vi "test BC + RTs.vi"(8 "error in":errorcluster, 11 "TestCase in":refnum<class "Create Execution Unit.lvclass">) -> (0 "error out":errorcluster, 3 "TestCase out":refnum<class "Create Execution Unit.lvclass">)   [LabVIEW 2020, in "Create Execution Unit.lvclass"]
uses:
  Create Execution Unit.lvclass
  C:/Program Files (x86)/National Instruments/LabVIEW 2020/vi.lib/addons/_JKI Toolkits/VI Tester/TestCase.llb/TestCase.lvclass
  Shared/Map of Messages to Value Indexes.ctl
  Shared/Message Map Key.ctl
  Engine/Implementation/Rx Execution Unit/Message Map Value.ctl
  Shared/Message Definition.ctl
  Shared/Message Type.ctl
  Shared/Terminal Endpoint.ctl
  Shared/Address.ctl
  Shared/Parameter Definition.ctl
  <vilib>/addons/_JKI Toolkits/VI Tester/TestCase.llb/TestCase.lvclass
  Scripting/AIM MIL-STD-1553 Scripting.lvlib
  Shared/Initialization Method.ctl
  Shared/Device Parameters.ctl
  Engine/Implementation/Execution Unit Factory/Execution Unit Factory.lvclass
  Engine/Implementation/Rx Execution Unit/Rx Execution Unit.lvclass
  Engine/Implementation/Shared Resources/Shared Resources.lvclass
  Shared/Data Word Format.ctl
  Engine/Custom Device/Logging Configuration.ctl
  Engine/Custom Device/Custom Device.lvlib
  Shared/Coupling Mode.ctl
  Shared/Bus Selection.ctl
  C:/dev/git/niveristand-custom-device-testing-tools/VeriStandScriptingTestCase/VeriStandScriptingTestCase.lvclass
  C:/dev/git/niveristand-aim-milStd1553-custom-device/Source/Custom Device Support/Tests/Unit/Create Execution Unit/Create Execution Unit.lvclass
  C:/dev/git/niveristand-aim-milStd1553-custom-device/Source/Custom Device Support/Engine/Implementation/Shared Resources/Shared Resources.lvclass
  C:/dev/git/niveristand-aim-milStd1553-custom-device/Source/Custom Device Support/Engine/Interfaces/Shared Resources/Shared Resources.lvclass
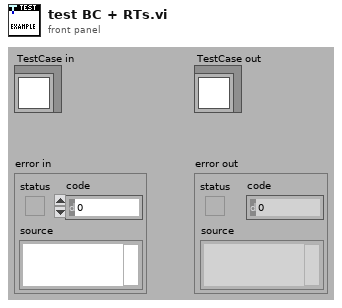
[diagram p1: front panel]
types:
  T1 = typedef "Map of Messages to Value Indexes.ctl" = map{T2, T3}
  T2 = typedef "Message Map Key.ctl" = cluster{"HW channel":u16, "terminal address":u16, "subaddress":u16, "mode code":u16}
  T3 = typedef "AIM MIL-STD-1553 Engine.lvlib/Implementation.lvlib/Rx Execution Unit.lvclass/Message Map Value.ctl" = cluster{"value indexes":i32[], "message":T4, "Tx status count":i32, "Rx status count":i32}
  T4 = typedef "Message Definition.ctl" = cluster{"name":string, "message type":T5, "endpoint Tx":T6, "endpoint Rx":T6, "create timestamp channel":bool, "mode code":u16, "number of words":u16, "parameters":cluster{"name":string, "default value":dbl, "unit":string, "parameter definition":T8}[]}
  T5 = typedef "Message Type.ctl" = string
  T6 = typedef "Terminal Endpoint.ctl" = cluster{"terminal address":T7, "subaddress":T7}
  T7 = typedef "Address.ctl" = u16
  T8 = typedef "Parameter Definition.ctl" = cluster{"start index":i32, "size (bits)":i32, "encoding":enum16{"BNR", "BCD", "Discrete"}, "signed":bool, "multiplier":dbl, "offset":dbl}
  T9 = typedef "Device Parameters.ctl" = cluster{"initialization method":T10, "card number":i32, "pxi slot number":i32, "biu number":i32, "bus selection":T11, "coupling mode":T12}
  T10 = typedef "Initialization Method.ctl" = enum16{"PXI Slot Number", "Card Number"}
  T11 = typedef "Bus Selection.ctl" = enum16{"Both", "Primary", "Secondary"}
  T12 = typedef "Coupling Mode.ctl" = enum16{"Isolated Onboard Termination", "Transformer Coupled", "Direct Coupled", "External with Onboard Termination", "Onboard Digital Wrap-around"}
  T13 = typedef "AIM MIL-STD-1553 Engine.lvlib/Custom Device.lvlib/Logging Configuration.ctl" = cluster{"configured":bool, "directory":string, "file name":string, "timestamp file name":bool, "data word format":T14}
  T14 = typedef "Data Word Format.ctl" = string
  T15 = typedef "Custom Device API.lvlib/Custom Device Item Ref.ctl" = u64
  T16 = typedef "AIM MIL-STD-1553 Engine.lvlib/Interfaces.lvlib/Execution Unit Information.ctl" = cluster{"Execution Unit":refnum<class "Execution Unit.lvclass">, "Incoming Channels":T15[], "Outgoing Channels":T15[], "ReadWrite Channels":T15[]}
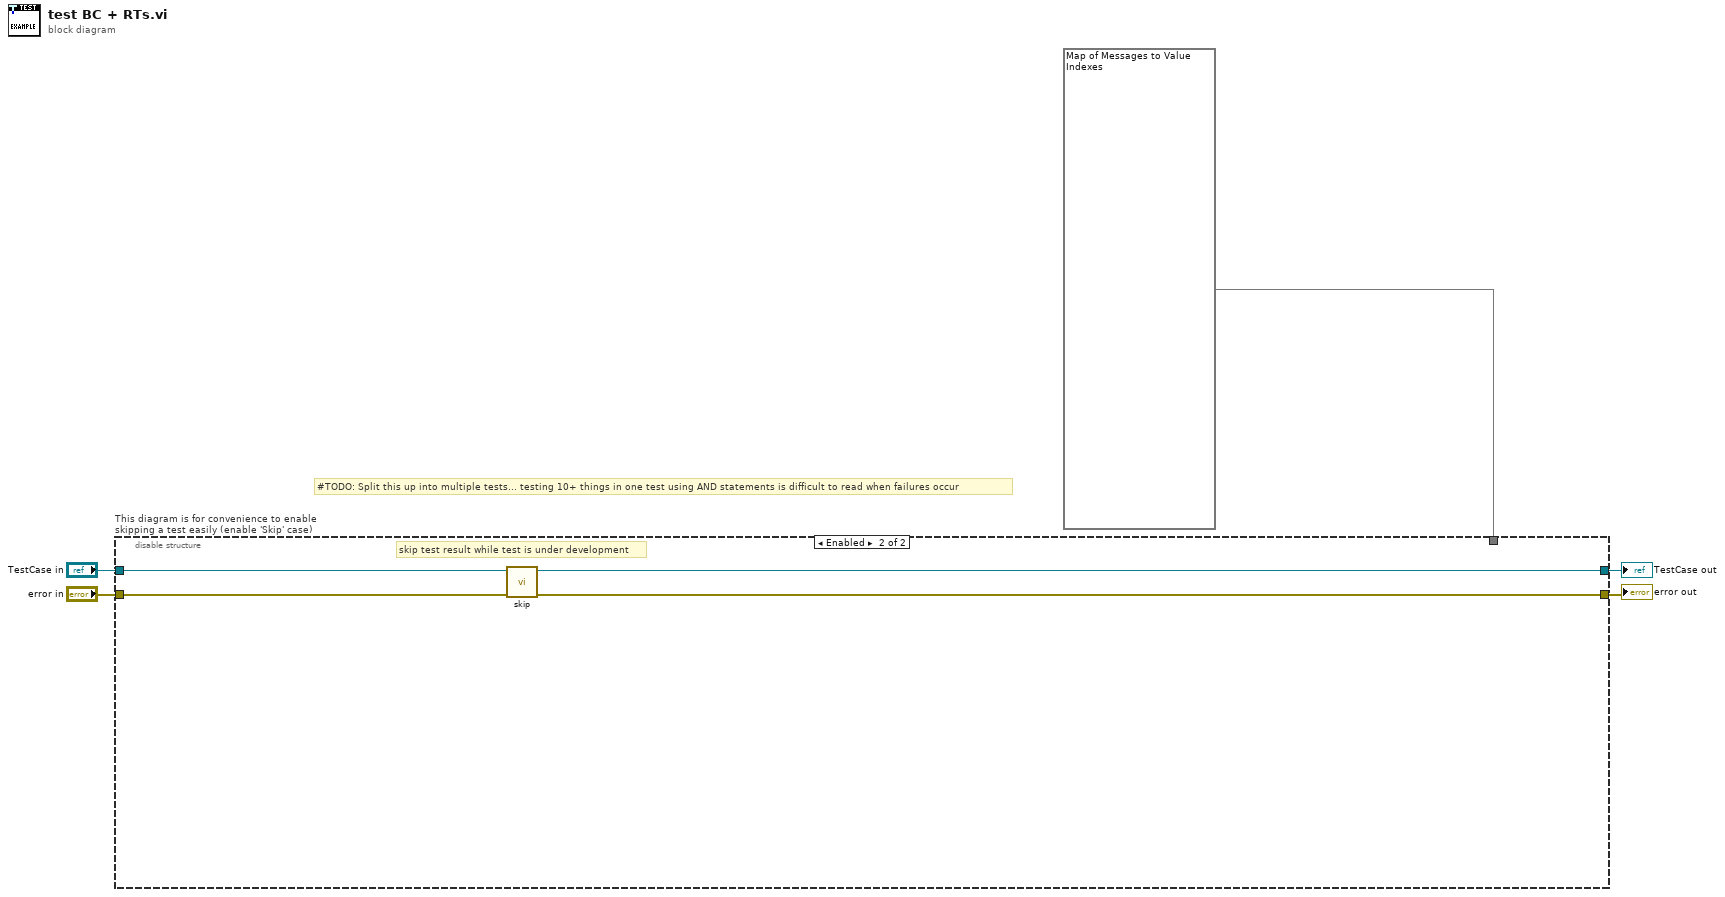
[diagram p0: block diagram]
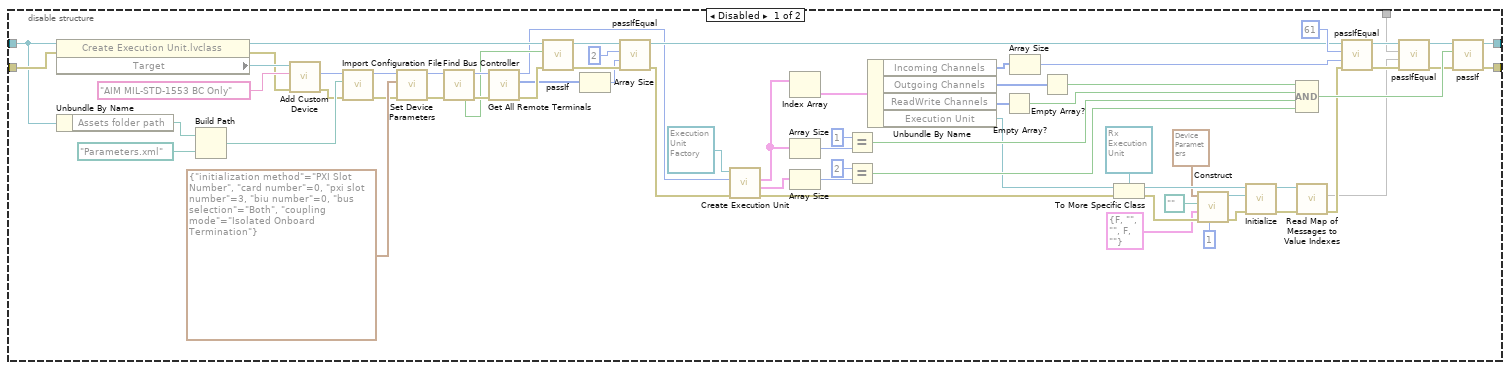
[diagram p2: hidden frame]
diagram:
  # "#TODO: Split this up into multiple tests... testing 10+ things in one test using AND statements is difficult to read when failures occur"
  n1 = disable-structure "This diagram is for convenience to enable skipping a test easily (enable 'Skip' case)" shown="Enabled" {
    disable-tunnel: "TestCase in" -> [w68 w77]
    disable-tunnel: [w34 w75] -> w2
    disable-tunnel: [w33 w76] -> w4
    disable-tunnel: "error in" -> [w72 w74]
    disable-tunnel: T1 {{"HW channel"=0, "terminal address"=1, "subaddress"=2, "mode code"=0}={"value indexes"=[0], "message"={"name"="BC to RT1 (SA2)", "message type"="BC to RT", "endpoint Tx"={"terminal address"=0, "subaddress"=0}, "endpoint Rx"={"terminal address"=1, "subaddress"=2}, "create timestamp channel"=TRUE, "mode code"=0, "number of words"=4, "parameters"=[{"name"="Word 00", "default value"=0.0, "unit"="", "parameter definition"={"start index"=0, "size (bits)"=16, "encoding"=enum."BNR", "signed"=FALSE, "multiplier"=1.0, "offset"=0.0}}, {"name"="Word 01", "default value"=0.0, "unit"="", "parameter definition"={"start index"=16, "size (bits)"=16, "encoding"=enum."BNR", "signed"=FALSE, "multiplier"=1.0, "offset"=0.0}}, {"name"="Word 02", "default value"=0.0, "unit"="", "parameter definition"={"start index"=32, "size (bits)"=16, "encoding"=enum."BNR", "signed"=FALSE, "multiplier"=1.0, "offset"=0.0}}, {"name"="Word 03", "default value"=0.0, "unit"="", "parameter definition"={"start index"=48, "size (bits)"=16, "encoding"=enum."BNR", "signed"=FALSE, "multiplier"=1.0, "offset"=0.0}}]}, "Tx status count"=0, "Rx status count"=1}, {"HW channel"=0, "terminal address"=1, "subaddress"=5, "mode code"=0}={"value indexes"=[16], "message"={"name"="RT1 to BC (SA5)", "message type"="RT to BC", "endpoint Tx"={"terminal address"=1, "subaddress"=5}, "endpoint Rx"={"terminal address"=0, "subaddress"=0}, "create timestamp channel"=TRUE, "mode code"=0, "number of words"=4, "parameters"=[{"name"="Word 00", "default value"=0.0, "unit"="", "parameter definition"={"start index"=0, "size (bits)"=16, "encoding"=enum."BNR", "signed"=FALSE, "multiplier"=1.0, "offset"=0.0}}, {"name"="Word 01", "default value"=0.0, "unit"="", "parameter definition"={"start index"=16, "size (bits)"=16, "encoding"=enum."BNR", "signed"=FALSE, "multiplier"=1.0, "offset"=0.0}}, {"name"="Word 02", "default value"=0.0, "unit"="", "parameter definition"={"start index"=32, "size (bits)"=16, "encoding"=enum."BNR", "signed"=FALSE, "multiplier"=1.0, "offset"=0.0}}, {"name"="Word 03", "default value"=0.0, "unit"="", "parameter definition"={"start index"=48, "size (bits)"=16, "encoding"=enum."BNR", "signed"=FALSE, "multiplier"=1.0, "offset"=0.0}}]}, "Tx status count"=1, "Rx status count"=0}, {"HW channel"=0, "terminal address"=1, "subaddress"=21, "mode code"=0}={"value indexes"=[40, 45], "message"={"name"="RT15 to RT1 (SA21)", "message type"="RT to RT", "endpoint Tx"={"terminal address"=15, "subaddress"=21}, "endpoint Rx"={"terminal address"=1, "subaddress"=21}, "create timestamp channel"=TRUE, "mode code"=0, "number of words"=4, "parameters"=[{"name"="Parameter 4", "default value"=0.0, "unit"="", "parameter definition"={"start index"=0, "size (bits)"=32, "encoding"=enum."BNR", "signed"=TRUE, "multiplier"=1.0, "offset"=0.0}}, {"name"="Parameter 5", "default value"=0.0, "unit"="", "parameter definition"={"start index"=32, "size (bits)"=32, "encoding"=enum."BNR", "signed"=FALSE, "multiplier"=1.0, "offset"=0.0}}]}, "Tx status count"=1, "Rx status count"=1}, {"HW channel"=0, "terminal address"=1, "subaddress"=31, "mode code"=16}={"value indexes"=[10], "message"={"name"="MC 16", "message type"="MC", "endpoint Tx"={"terminal address"=1, "subaddress"=31}, "endpoint Rx"={"terminal address"=0, "subaddress"=0}, "create timestamp channel"=TRUE, "mode code"=16, "number of words"=1, "parameters"=[{"name"="Word 00", "default value"=0.0, "unit"="", "parameter definition"={"start index"=0, "size (bits)"=16, "encoding"=enum."BNR", "signed"=FALSE, "multiplier"=1.0, "offset"=0.0}}]}, "Tx status count"=1, "Rx status count"=0}, {"HW channel"=0, "terminal address"=1, "subaddress"=31, "mode code"=17}={"value indexes"=[13], "message"={"name"="MC 17", "message type"="MC", "endpoint Tx"={"terminal address"=0, "subaddress"=0}, "endpoint Rx"={"terminal address"=1, "subaddress"=31}, "create timestamp channel"=TRUE, "mode code"=17, "number of words"=1, "parameters"=[{"name"="Word 00", "default value"=0.0, "unit"="", "parameter definition"={"start index"=0, "size (bits)"=16, "encoding"=enum."BNR", "signed"=FALSE, "multiplier"=1.0, "offset"=0.0}}]}, "Tx status count"=0, "Rx status count"=1}, {"HW channel"=0, "terminal address"=15, "subaddress"=3, "mode code"=0}={"value indexes"=[6], "message"={"name"="BC to RT15 (SA3)", "message type"="BC to RT", "endpoint Tx"={"terminal address"=0, "subaddress"=0}, "endpoint Rx"={"terminal address"=15, "subaddress"=3}, "create timestamp channel"=TRUE, "mode code"=0, "number of words"=4, "parameters"=[{"name"="Parameter 0", "default value"=0.0, "unit"="", "parameter definition"={"start index"=0, "size (bits)"=32, "encoding"=enum."BNR", "signed"=TRUE, "multiplier"=1.0, "offset"=0.0}}, {"name"="Parameter 1", "default value"=0.0, "unit"="", "parameter definition"={"start index"=32, "size (bits)"=32, "encoding"=enum."BNR", "signed"=FALSE, "multiplier"=1.0, "offset"=0.0}}]}, "Tx status count"=0, "Rx status count"=1}, {"HW channel"=0, "terminal address"=15, "subaddress"=6, "mode code"=0}={"value indexes"=[36], "message"={"name"="RT15 to BC (SA6)", "message type"="RT to BC", "endpoint Tx"={"terminal address"=15, "subaddress"=6}, "endpoint Rx"={"terminal address"=0, "subaddress"=0}, "create timestamp channel"=TRUE, "mode code"=0, "number of words"=4, "parameters"=[{"name"="Parameter 2", "default value"=0.0, "unit"="", "parameter definition"={"start index"=0, "size (bits)"=32, "encoding"=enum."BNR", "signed"=TRUE, "multiplier"=1.0, "offset"=0.0}}, {"name"="Parameter 3", "default value"=0.0, "unit"="", "parameter definition"={"start index"=32, "size (bits)"=32, "encoding"=enum."BNR", "signed"=FALSE, "multiplier"=1.0, "offset"=0.0}}]}, "Tx status count"=1, "Rx status count"=0}, {"HW channel"=0, "terminal address"=15, "subaddress"=20, "mode code"=0}={"value indexes"=[22, 29], "message"={"name"="RT1 to RT15 (SA20)", "message type"="RT to RT", "endpoint Tx"={"terminal address"=1, "subaddress"=20}, "endpoint Rx"={"terminal address"=15, "subaddress"=20}, "create timestamp channel"=TRUE, "mode code"=0, "number of words"=4, "parameters"=[{"name"="Word 00", "default value"=0.0, "unit"="", "parameter definition"={"start index"=0, "size (bits)"=16, "encoding"=enum."BNR", "signed"=FALSE, "multiplier"=1.0, "offset"=0.0}}, {"name"="Word 01", "default value"=0.0, "unit"="", "parameter definition"={"start index"=16, "size (bits)"=16, "encoding"=enum."BNR", "signed"=FALSE, "multiplier"=1.0, "offset"=0.0}}, {"name"="Word 02", "default value"=0.0, "unit"="", "parameter definition"={"start index"=32, "size (bits)"=16, "encoding"=enum."BNR", "signed"=FALSE, "multiplier"=1.0, "offset"=0.0}}, {"name"="Word 03", "default value"=0.0, "unit"="", "parameter definition"={"start index"=48, "size (bits)"=16, "encoding"=enum."BNR", "signed"=FALSE, "multiplier"=1.0, "offset"=0.0}}]}, "Tx status count"=1, "Rx status count"=1}} ("map of messages to value indexes") -> [w15 _]
    frame Disabled {
      n2 = property class="Create Execution Unit.lvclass"(reference=w68, error in=w72) -> (reference out=w73:refnum<class "Create Execution Unit.lvclass">, error out=w69:errorcluster, "Target"=w70:refnum<k24>)
      n3 = Unbundle By Name(w68) -> ("Assets folder path"=w67:path)
      n4 = Build Path(base path=w67, name or relative path=path "Parameters.xml") -> (appended path=w65:path)
      n5 = call "Add Custom Device.vi"("error in"=w69, "custom device name"="AIM MIL-STD-1553 BC Only" ("name"), "target"=w70) -> ("error out"=w6:errorcluster, "custom device ref out"=w7:T15)  [unwired: 6 in, 1 out]
      n6 = call "Import Configuration File.vi"("error in"=w6, "parameters configuration file path"=w65, "custom device ref"=w7) -> ("error out"=w62:errorcluster, "custom device ref out"=w64:T15)  [unwired: 7 in]
      n7 = call "Set Device Parameters.vi"("error in"=w62, "device parameters"=T9 {"initialization method"=enum."PXI Slot Number", "card number"=0, "pxi slot number"=3, "biu number"=0, "bus selection"=enum."Both", "coupling mode"=enum."Isolated Onboard Termination"}, "custom device"=w64) -> ("error out"=w50:errorcluster, "custom device out"=w52:T15)  [unwired: 7 in]
      n8 = call "Find Bus Controller.vi"("error in"=w50, "port in"=w52) -> ("error out"=w49:errorcluster, "port out"=w51:T15, "found?"=w48:bool)  [unwired: 6 in, 1 out]
      n9 = call "Get All Remote Terminals.vi"("error in"=w49, "port in"=w51) -> ("error out"=w47:errorcluster, "remote terminals"=w46:T15[], "port out"=w13:T15)  [unwired: 7 in]
      n10 = call-dynamic "passIf.vi"("error in (no error)"=w47, "pass"=w48, "TestCase in"=w73) -> ("error out"=w54:errorcluster, "TestCase out"=w55:refnum<class "Create Execution Unit.lvclass">)  [unwired: 7 in]
      n11 = Array Size(array=w46) -> (size(s)=w45:i32)
      n12 = call-dynamic "passIfEqual.vi"("error in (no error)"=w54, "y"=w45, "x"=2 ("size(s)"), "TestCase in"=w55) -> ("error out"=w53:errorcluster, "TestCase out"=w37:refnum<class "Create Execution Unit.lvclass">)  [unwired: 6 in]
      n13 = call-dynamic "Create Execution Unit.vi"("error in"=w53, "custom device ref"=w13, "execution unit factory"=refnum<class "Execution Unit Factory.lvclass"> refnum ("Execution Unit Factory Implementation in")) -> ("error out"=w27:errorcluster, "asynchronous execution units"=w60:T16[], "inline execution units"=w43:T16[])  [unwired: 5 in, 1 out]
      n14 = Index Array(array=w43) -> (element=w42:T16)  [unwired: 1 in]
      n15 = Array Size(array=w43) -> (size(s)=w59:i32)
      n16 = Array Size(array=w60) -> (size(s)=w58:i32)
      n17 = Equal?(x=1, y=w59) -> (x = y?=w36:bool)
      n18 = Equal?(x=2, y=w58) -> (x = y?=w35:bool)
      n19 = Unbundle By Name(w42) -> ("Incoming Channels"=w41:T15[], "Outgoing Channels"=w11:T15[], "ReadWrite Channels"=w9:T15[], "Execution Unit"=w28:refnum<class "Execution Unit.lvclass">)
      n20 = Empty Array?(array=w9) -> (empty?=w8:bool)
      n21 = Array Size(array=w41) -> (size(s)=w39:i32)
      n22 = Empty Array?(array=w11) -> (empty?=w10:bool)
      n23 = To More Specific Class(target class=refnum<class "Rx Execution Unit.lvclass"> refnum ("Rx execution unit in"), reference=w28, error in=w27) -> (specific class reference=w29:refnum<class "Rx Execution Unit.lvclass">, error out=w24:errorcluster)
      n24 = call "Construct.vi"(6:1 ("number of ports"), "error in"=w24, "logging configuration"=T13 {"configured"=FALSE, "directory"="", "file name"="", "timestamp file name"=FALSE, "data word format"=""}, "1553 configuration"=path "" ("hardware config file"), "device parameters"=T9 {"initialization method"=enum."PXI Slot Number", "card number"=0, "pxi slot number"=0, "biu number"=0, "bus selection"=enum."Both", "coupling mode"=enum."Isolated Onboard Termination"}) -> ("error out"=w23:errorcluster, "shared resources out"=w26:refnum<class "Shared Resources.lvclass">)  [unwired: 5 in]
      n25 = call-dynamic "Initialize.vi"("error in"=w23, "shared resources"=w26, "Rx Execution Unit Implementation in"=w29) -> ("error out"=w12:errorcluster, "Rx Execution Unit Implementation out"=w30:refnum<class "Rx Execution Unit.lvclass">)  [unwired: 7 in]
      n26 = Compound Arithmetic op=AND(w10, w8, w36, w35) -> (w40:bool)
      n27 = call "Read Map of Messages to Value Indexes.vi"("error in"=w12, "Rx execution unit in"=w30) -> ("error out"=w31:errorcluster, "map of messages to value indexes"=w14:T1)  [unwired: 7 in, 1 out]
      n28 = call-dynamic "passIfEqual.vi"("error in (no error)"=w31, "y"=w39, "x"=61 ("size(s)"), "TestCase in"=w37) -> ("error out"=w19:errorcluster, "TestCase out"=w18:refnum<class "Create Execution Unit.lvclass">)  [unwired: 6 in]
      n29 = call-dynamic "passIfEqual.vi"("error in (no error)"=w19, "y"=w14, "x"=w15, "TestCase in"=w18) -> ("error out"=w16:errorcluster, "TestCase out"=w17:refnum<class "Create Execution Unit.lvclass">)  [unwired: 6 in]
      n30 = call-dynamic "passIf.vi"("error in (no error)"=w16, "pass"=w40, "TestCase in"=w17) -> ("error out"=w33:errorcluster, "TestCase out"=w34:refnum<class "Create Execution Unit.lvclass">)  [unwired: 7 in]
    }
    frame Enabled {
      # "skip test result while test is under development"
      n31 = call <vilib>:"skip.vi"("error in (no error)"=w74, "TestCase in"=w77) -> ("error out"=w76:errorcluster, "TestCase out"=w75:refnum<class "Create Execution Unit.lvclass">)  [unwired: 8 in]
    }
  }
  "error out" <- w4
  "TestCase out" <- w2
